vi "dequeue display queues.vi"(8 "error in":errorcluster) -> (0 "error out":errorcluster, 2 "Empty?":bool, 3 "data out":sgl[](array[numeric]))   [LabVIEW 2018]
uses:
  Controls/Queue Manager Actions.ctl
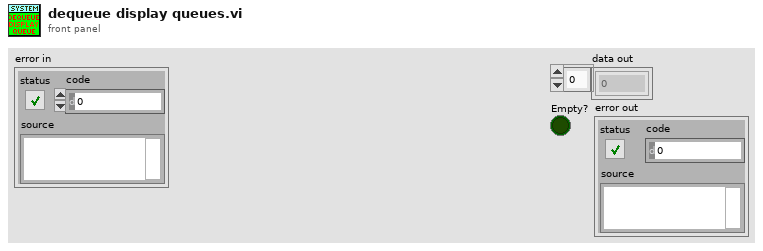
[diagram p1: front panel]
types:
  T1 = typedef "Queue Manager Actions.ctl" = enum16{"Init", "Enqueue", "Enqueue All", "Preview Queue", "Dequeue", "Get Status", "Flush Queue", "Flush All Queues", "Release All Queues", "Release Queue", "Enqueue at Opposite End"}
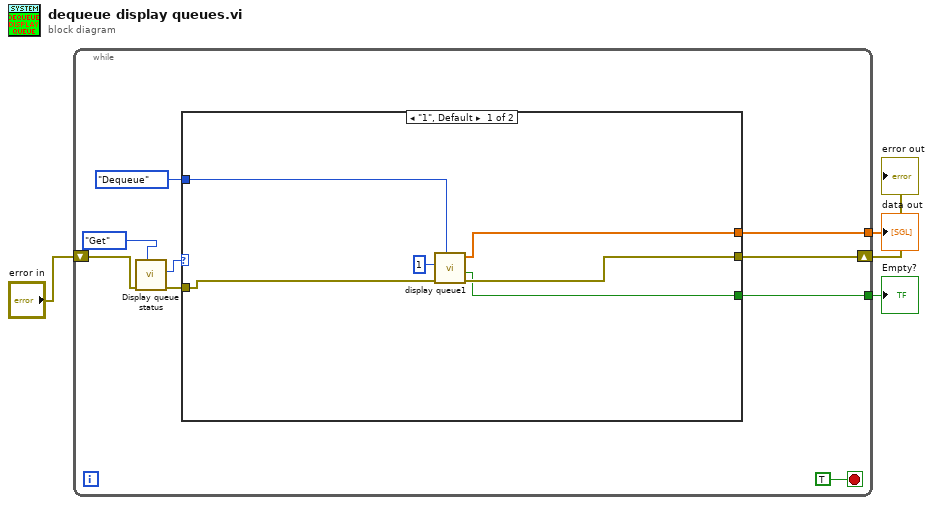
[diagram p0: block diagram]
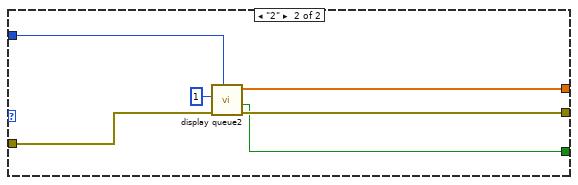
[diagram p2: hidden frame]
diagram:
  n1 = while {
    tunnel: [w7] -> w3
    shift-right: [w6] -> w1
    shift-left: "error in" -> [w12]
    tunnel: [w5] -> w2
    stop <- TRUE stop-if-true
    n2 = call "Display queue status.vi"("action"=enum16{"Init", "Get", "Set"}."Get", "error in"=w12) -> ("error out"=w9:errorcluster, "dequeue channel out"=w10:enum16{"1", "2"})  [unwired: 6 in, 1 out]
    n3 = case shown="\"1\", Default" w10 {
      tunnel: w9 -> [w19 w25]
      tunnel: Queue_Manager_Actions."Dequeue" ("Action") -> [w17 w24]
      tunnel: [w16 w23] -> w7
      tunnel: [w15 w22] -> w6
      tunnel: [w14 w21] -> w5
      frame "1", Default {
        n4 = call "display queue1.vi"("Action"=w17, "error in (no error)"=w19, "timeout in ms (-1)"=1) -> ("error out"=w15:errorcluster, "Empty?"=w14:bool, "data out"=w16:sgl[])  [unwired: 5 in, 1 out]
      }
      frame "2" {
        n5 = call "display queue2.vi"("Action"=w24, "error in (no error)"=w25, "timeout in ms (-1)"=1) -> ("error out"=w22:errorcluster, "Empty?"=w21:bool, "data out"=w23:sgl[])  [unwired: 5 in, 1 out]
      }
    }
  }
  "data out" <- w3
  "Empty?" <- w2
  "error out" <- w1
